vi "Get End of Last Record.vi"(9 "Offset in":i32, 10 "Bytes in":u8[](array[numeric]) format="%.0x", 11 "pcap_Parse_Build_CIF":refnum<class "pcap_Parse_Build_CIF.lvclass">) -> (2 "End Offset":i32)   [LabVIEW 2021, in "pcap_Parse_Build_CIF.lvclass"]
uses:
  pcap_Parse_Build_CIF.lvclass
  pcap_Parse_Build_CIF.lvclass/pcap_Parse_Build_CIF.ctl
  <vilib>/CIF Foundation/CIF Utilities/DataTypes/DataTypes_CIF_U.lvlib
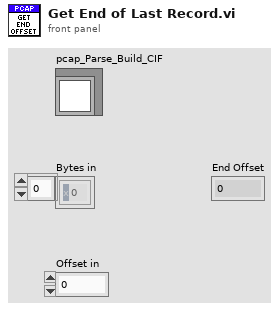
[diagram p1: front panel]
types:
  T1 = typedef "DataTypes_CIF_U.lvlib/Endian.ctl" = enum16{"Little Endian", "Big Endian"}
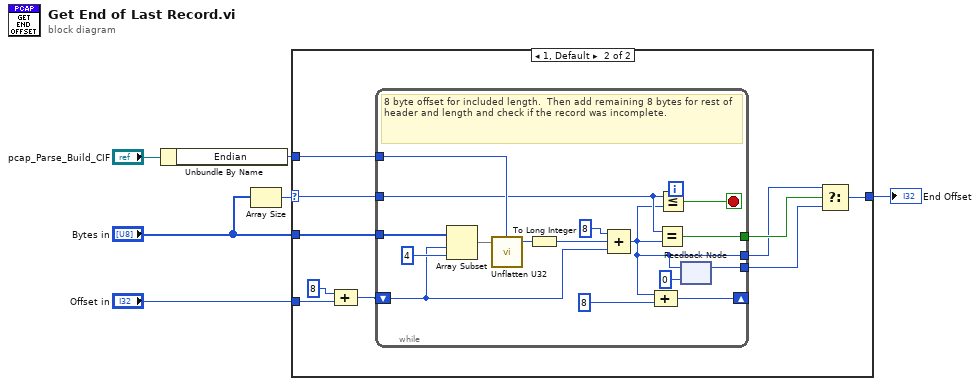
[diagram p0: block diagram]
diagram:
  n1 = Unbundle By Name("pcap_Parse_Build_CIF") -> ("Endian"=w3:T1)
  n2 = Array Size(array="Bytes in") -> (size(s)=w2:i32)
  n3 = case shown="1, Default" w2 {
    selector: w2 -> [w7 w15]
    tunnel: "Bytes in" -> [_ w17]
    tunnel: [w7 w10] -> w4
    tunnel: w3 -> [_ w16]
    tunnel: "Offset in" -> [_ w12]
    frame 0 {
    }
    frame 1, Default {
      n4 = Compound Arithmetic op=ADD(8 ("Offset"), w12) -> (w13:i32)
      n5 = while {
        tunnel: w15 -> [w22]
        tunnel: w17 -> [w30]
        shift-right: [w24] -> _
        shift-left: w13 -> [w23]
        tunnel: w16 -> [w27]
        tunnel: [w21] -> w11
        tunnel: [w20] -> w9
        tunnel: [w18] -> w8
        stop <- w33 stop-if-true
        # "8 byte offset for included length.  Then add remaining 8 bytes for rest of header and length and check if the record was incomplete."
        n6 = Array Subset(array=w30, index=w23, length=4 ("index")) -> (w31:u8[])
        n7 = call <vilib>:"Unflatten U32.vi"("Flat Data"=w31, "Endian"=w27) -> ("U32"=w29:u32)  [unwired: 3 in]
        n8 = To Long Integer(number=w29) -> (32bit integer=w28:i32)
        n9 = Compound Arithmetic op=ADD(8 ("value"), w28, w23) -> (w20:i32)
        n10 = Compound Arithmetic op=ADD(w20, 8 ("value")) -> (w24:i32)
        n11 = Equal?(x=w22, y=w20) -> (x = y?=w21:bool)
        n12 = Less Or Equal?(x=w22, y=w20) -> (x <= y?=w33:bool)
        n13 = feedback-in #1(w20) -> ()
        n14 = feedback #1(0) -> (w18:i32)
      }
      n15 = Select(t=w9, s=w11, f=w8) -> (s? t:f=w10:i32)
    }
  }
  "End Offset" <- w4
